vi "Parse Repo Details.vi"(8 "error in (no error)":errorcluster, 10 "Repo file in":T1, 11 "Repo in":refnum<class "Repo.lvclass">) -> (0 "error out":errorcluster, 2 "Repo file out":T1, 3 "Repo out":refnum<class "Repo.lvclass">)   [LabVIEW 2016, in "Packages.lvlib" / "VIPM.lvlib"]
uses:
  VIPM.lvlib
  Repo_class/Repo.lvclass
  <vilib>/Utility/config.llb/Config Data RefNum.ctl
  Repo_class/Repo.lvclass/Repo.ctl
  Repo_class/Write Name.vi
  Repo_class/Write LastUpdated.vi
  <vilib>/Utility/config.llb/Read Key (String).vi
  <vilib>/Utility/config.llb/NI_LVConfig.lvlib
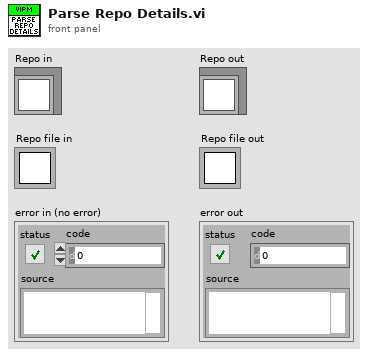
[diagram p1: front panel]
types:
  T1 = typedef "NI_LVConfig.lvlib/Config Data RefNum.ctl" = refnum<k1>
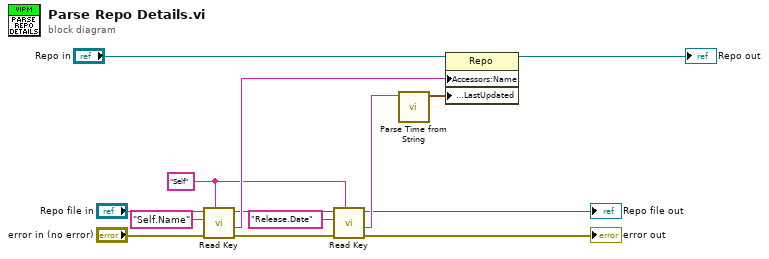
[diagram p0: block diagram]
diagram:
  w9 = "Self" ("section")
  n1 = call-poly <vilib>:"Read Key.vi"("section"=w9, "error in (no error)"="error in (no error)", "key"="Self.Name", "refnum"="Repo file in") -> ("error out"=w6:errorcluster, "value"=w11:string, "refnum out"=w5:T1)  [unwired: 4 in, 1 out]
  n2 = call-poly <vilib>:"Read Key.vi"("section"=w9, "error in (no error)"=w6, "key"="Release.Date", "refnum"=w5) -> ("error out"=→"error out":errorcluster, "value"=w12:string, "refnum out"=→"Repo file out":T1)  [unwired: 4 in, 1 out]
  n3 = call "Parse Time from String.vi"("Time string"=w12) -> ("Timestamp"=w13:timestamp)  [unwired: 10 in]
  n4 = property class="Repo"(reference="Repo in", "Accessors:Name"=w11, "Accessors:LastUpdated"=w13) -> (reference out=→"Repo out":refnum<class "Repo.lvclass">)  [unwired: 1 in, 1 out]
